vi "GUMSSequenceGenerator.vi"() -> ()   [LabVIEW 2011]
uses:
  gumLV8p2/D/Labviewsoft/transport/GUMS/Kelvinox drivers/ITCAPPS - Copie.LLB/ITCSignal.ctl
  gumLV8p2/D/Labviewsoft/transport/GUMS/Kelvinox drivers/ITCAPPS - Copie.LLB/ITCSignals.ctl
  DAC/Visa name1.vi
  GlobalVar.vi
  stopButton.vi
  monochromatorcontrol/perHandlemonochromator.vi
  users/nicolas/PHySpec-SDK-1.0.0/Labview-example/libPhyspec/libPhyspec.lvlib
panel:
  out "counter 2":i32
  out "DMMX":string[][](array[string])
  out "Bloop gen":u32
  out "WVlenloop gen":u32
  out "Tloop gen":u32
  out "loopchange":u32
  out "DACindic":bool
  in  "Gain Cluster 2":T1={"Vsd"="DAC 1", "I 2probe 2"="DMM1", "Vxy"="Lockin2 X", "Vxx"="DMM2", "I leak BG"="I K2400_01", "I leak TG"="I K2400_02", "I Gain 1"=1000000.0, "V Gain 1"=1.0, "conversion factor BG"=1.0, "Vin / Vout 1"=1.0, "V Gain 2"=1.0, "Vin / Vout 2"=1.0, "V Gain 3"=1.0, "Vin / Vout 3"=1.0, "I Gain 2"=1.0, "I Gain 3"=1.0, "V BG"="V K2400_01", "V TG"="V K2400_02", "conversion factor TG"=1.0, "Vin / Vout 4"=1.0, "Vin / Vout 5"=1.0, "Manual Gain 1"=1.0, "Manual Gain 2"=1.0, "Manual Gain 3"=1.0} {"conversion factor TG" items=["1 V/V"=1.0, "4 V/V"=4.0, "15 V/V"=15.0, "30 V/V"=30.0, "45 V/V"=45.0]; "I Gain 3" items=["1"=1.0, "10"=10.0, "100"=100.0, "1K"=1000.0, "10K"=10000.0, "100K"=100000.0, "1M"=1000000.0, "10M"=10000000.0, "100M"=100000000.0, "1G"=1000000000.0]; "I Gain 2" items=["1"=1.0, "10"=10.0, "100"=100.0, "1K"=1000.0, "10K"=10000.0, "100K"=100000.0, "1M"=1000000.0, "10M"=10000000.0, "100M"=100000000.0, "1G"=1000000000.0]; "V Gain 3" items=["1"=1.0, "10"=10.0, "100"=100.0, "1K"=1000.0, "10K"=10000.0]; "V Gain 2" items=["1"=1.0, "10"=10.0, "100"=100.0, "1K"=1000.0, "10K"=10000.0]; "conversion factor BG" items=["1 V/V"=1.0, "4 V/V"=4.0, "15 V/V"=15.0, "30 V/V"=30.0, "45 V/V"=45.0]; "V Gain 1" items=["1"=1.0, "10"=10.0, "100"=100.0, "1K"=1000.0, "10K"=10000.0]; "I Gain 1" items=["1"=1.0, "10"=10.0, "100"=100.0, "1K"=1000.0, "10K"=10000.0, "100K"=100000.0, "1M"=1000000.0, "10M"=10000000.0, "100M"=100000000.0, "1G"=1000000000.0]}
  in  "EmptyAllArrays":bool
  in  "Sweep back to zero":bool
  out "counter":i32
  out "Num elements in col":i32[](array[numeric])
  out "Current col":i32
  in  "Refresh Rate [ms]":i32=1000 min=0
  out "Current sweep":dbl
  out "ITC ref":T2={"ITC"=0, "Signal"=enum."Sensor 3"}
  in  "Cancel run":bool
  out "DAC":refnum<visa-resource-name>
  out "K2400 2":refnum<visa-resource-name>
  out "Lockin1":refnum<visa-resource-name>
  out "K2400 1":refnum<visa-resource-name>
  out "Total sweep sequence":dbl[][](array[numeric])
  in  "Device Cluster":T4={"K2400 1"="", "K2400_1"=FALSE, "K2400 2"="", "K2400_2"=FALSE, "Lockin1"="", "Lockin1 present"=FALSE, "Lockin2"="", "Lockin2 present"=FALSE, "TIC"="", "Tcontrol"="OFF", "DAC"="", "DAC present"=FALSE, "Bfield query"=FALSE, "Wvlen query"=FALSE, "ITC signal"={"ITC"=0, "Signal"=enum."Sensor 1"}, "DMMX"=[["DMM1", ""]]}
  in  "Tab Control":T5(tab)
  in  "Sweep Toothsaw":bool
  in  "Loop Cluster":T6
  in  "START":bool
  in  "genTotalSequence":bool
  out "row state":i32[](array[numeric])
  out "Priority type array":string[](array[string])
  out "TotalPnts":dbl
  in  "Sweep back\nto zero?":bool
  in  "Conversion Factor Fix\n1 V = ??":dbl=1.0
  in  "Fix type":string(combo)
  in  "Sweep Bias":dbl[](array[numeric])
  in  "Fix Bias":dbl[](array[numeric])
  in  "Priority sweep":i32=2
  in  "Priority fix":i32=2
  in  "sweep start [V]":dbl=-1.0 min=-200.0 max=200.0
  in  "sweep stop [V]":dbl=-5.0 min=-250.0 max=250.0
  in  "Nb steps":i32=800
  in  "sweep stop 2 [V]":dbl min=-250.0 max=250.0
  in  "Nb steps 2":i32
  in  "Nb Sweep":i32=1
  in  "Nb steps fix2":i32
  in  "Fix stop 2":dbl min=-250.0 max=250.0
  in  "Nb steps fix":i32=800
  in  "Fix stop":dbl=-5.0 min=-250.0 max=250.0
  in  "Fix start":dbl=-1.0 min=-200.0 max=200.0
  in  "genSweepArray":bool
  in  "genFixArray":bool
  in  "Sweep Instrument":string(combo)
  in  "Conversion Factor Sweep\n1 V = ??":dbl=1.0
  in  "Fix Instrument":string(combo)
  in  "Sweep type":string(combo)
  in  "V step K2400 [V]":dbl=0.001
  in  "genSweepArray sweeploop":bool
  in  "genfixArray fixlooop simple":bool
  in  "T [K]":dbl[](array[numeric])
  in  "Priority T":i32=2
  in  "Nb T steps":i32=800
  in  "T stop [K]":dbl=-1.0 min=-200.0 max=200.0
  in  "T start [K]":dbl=-1.0 min=-200.0 max=200.0
  in  "genTarray":bool
  in  "Add T points":bool
  in  "Zero ramp Rate [T/min] 2":dbl=0.2 min=-200.0 max=200.0
  in  "Sweep Field back to zero":bool
  in  "B [T]":dbl[](array[numeric])
  in  "Priority B":i32=2
  in  "B start [T]":dbl=-1.0 min=-200.0 max=200.0
  in  "B stop [T]":dbl=-1.0 min=-200.0 max=200.0
  in  "Sweep Rate [T/min]":dbl=0.1 min=-200.0 max=200.0
  in  "Nb B steps":i32=800
  in  "GenBarray":bool
  in  "Add B points":bool
  in  "Set Persistent":bool=TRUE
  in  "Power stabilization":bool=TRUE
  in  "Wvlen Start [nm]":dbl=400.0
  in  "Wavelength [nm]":dbl[](array[numeric])
  in  "genWVLEN array":bool
  in  "Add wvlen points":bool
  in  "Nb Wvlen steps":i32=350
  in  "Wvlen stop [nm]":dbl=1100.0
  out "Laser Power [W]":dbl format="%#.2g"
  in  "START FC":bool
  out "Field ok !":bool
  in  "Bipolar":bool
  in  "High T (K)":dbl
  in  "Temperature Up rate (K/min)":dbl
  in  "Waiting time (min)":dbl
  in  "Base T (K)":dbl
  in  "sweep rate B (T/min)":dbl
  in  "Cooling field (T)":dbl
  out "I am":string
  in  "File Basename":string
  out "Bias factor":dbl
  in  "SD bias [V]":dbl=-1.0 min=-200.0 max=200.0
  in  "Nb steps Increase 2":dbl=10.0
  in  "Gate Increase 2 (V)":dbl=0.1
  in  "Nb steps Increase":dbl=10.0
  in  "Gate Increase (V)":dbl=-0.1
  out "x .or. y?":bool
  in  "Step Delay (ms)":dbl=1000.0
  out "Total Progress":dbl(slide) scale=0.0..1.0
  in  "Nb Loop":i32
  out "Nb Loop Indicator":i32=2
  out "Nb Sweep Indicator":i32=3
  out "conversion factor sweep":dbl(ring)=1.0 items=["1 V/V"=1.0, "4 V/V"=4.0, "15 V/V"=15.0, "30 V/V"=30.0, "45 V/V"=45.0]
  in  "stop":bool
  in  "V step [V]":dbl=0.001
  in  "Folder Name":path=path "D:/users/marc/20180122_LiIon_EL/Freezing02/OutputHighT002p2.dat"
  # "Magnetic Field"
  # "Wavelength"
  # "IV Sweep Setting"
  # "IV Fix Setting"
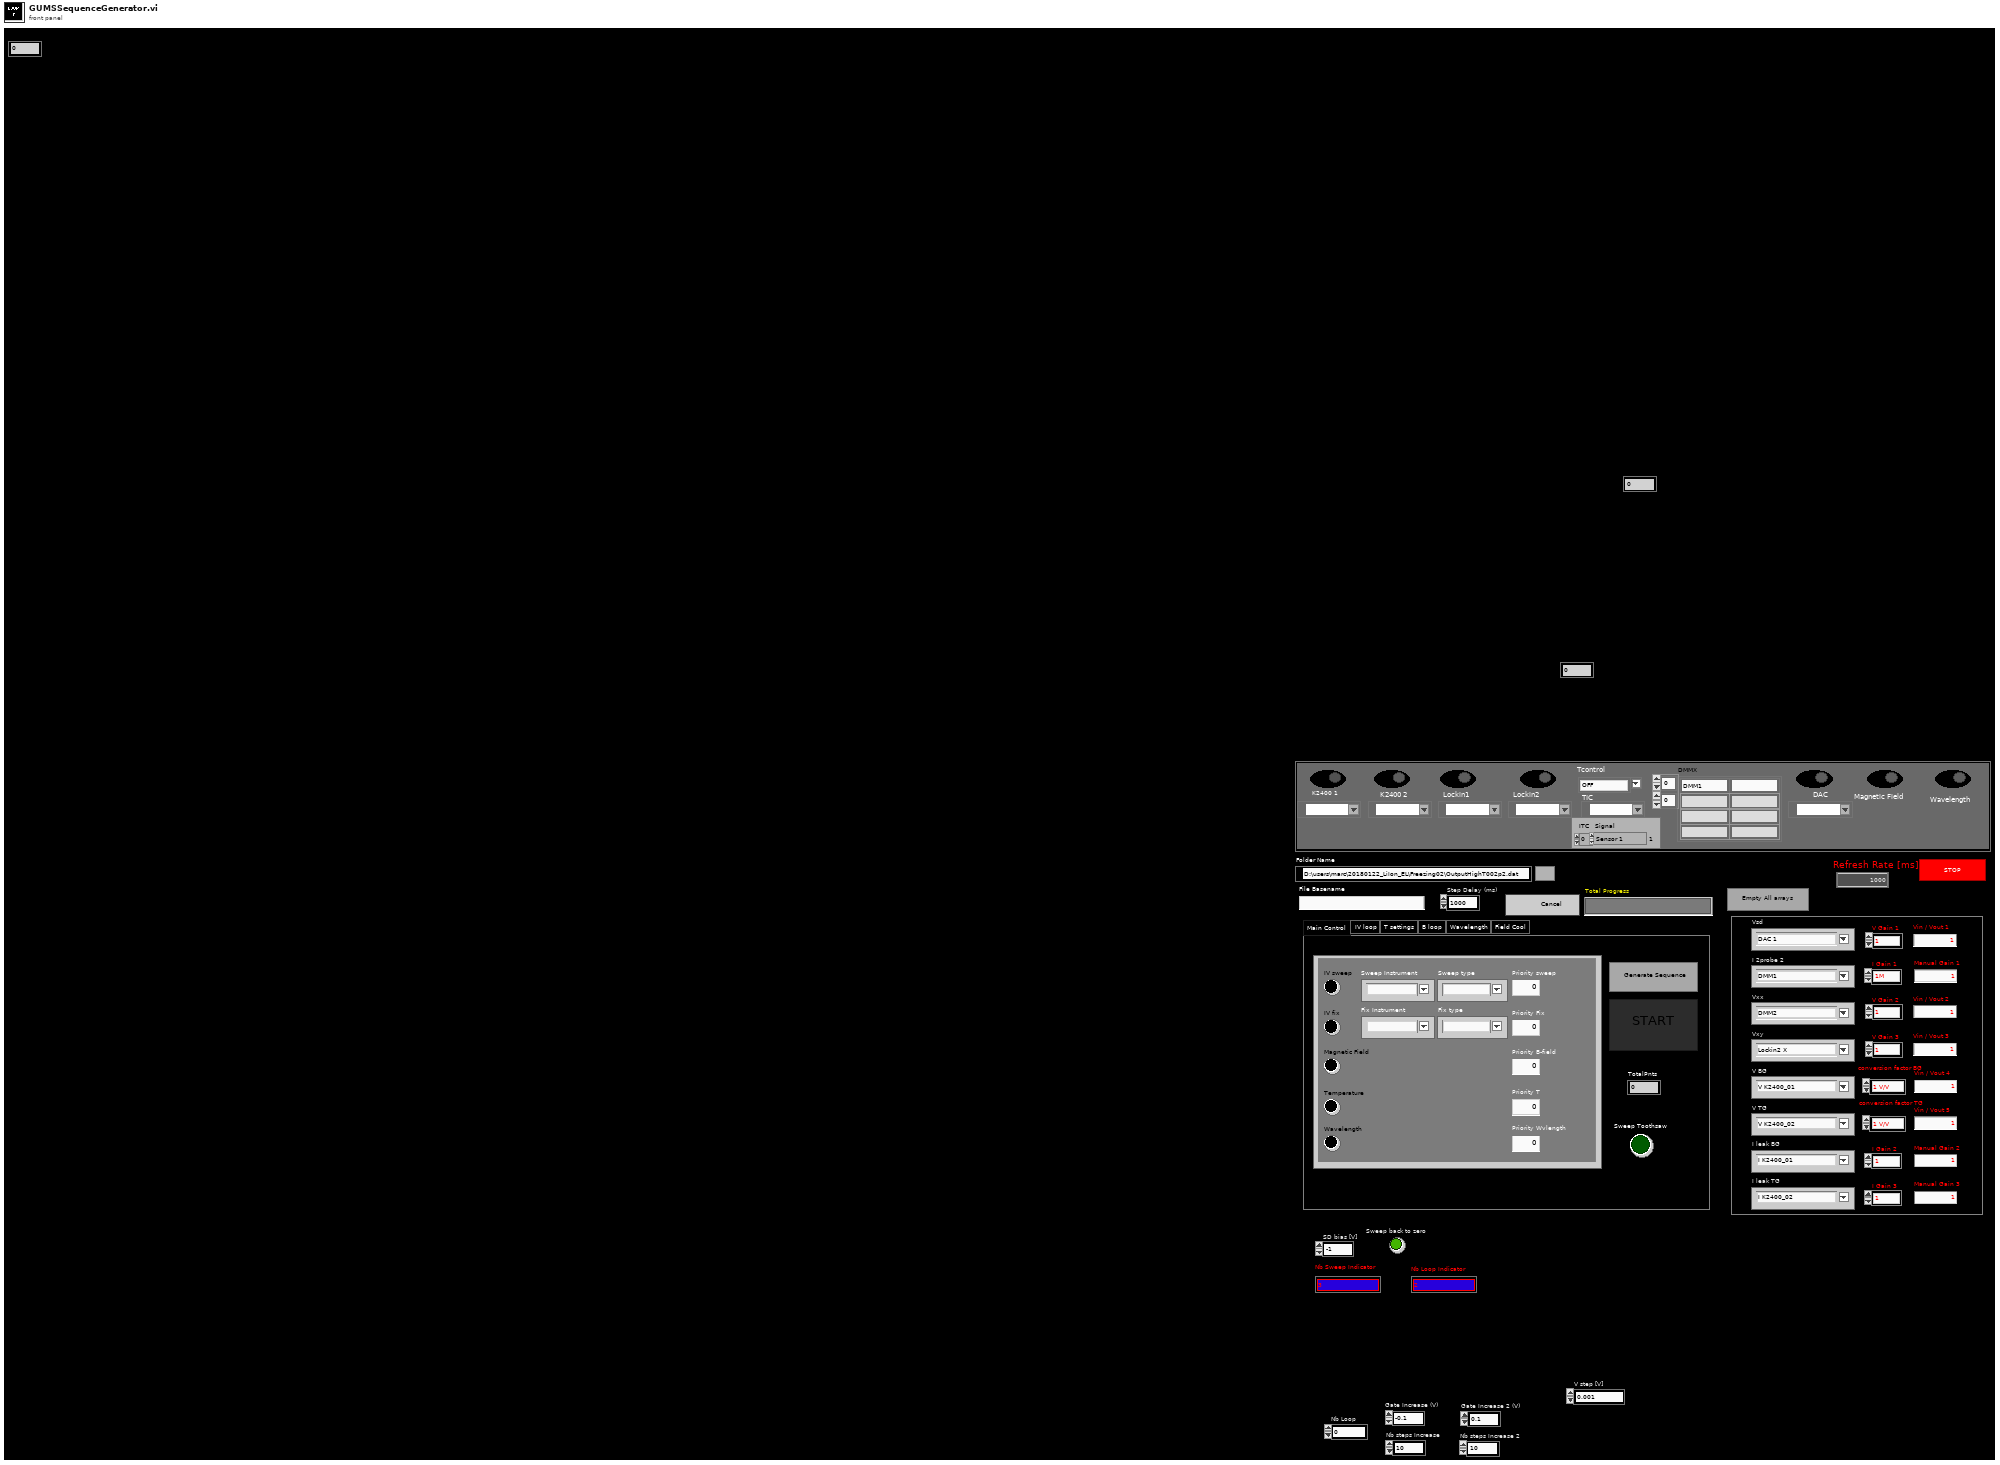
[diagram p1: front panel]
types:
  T1 = cluster{"Vsd":string, "I 2probe 2":string, "Vxy":string, "Vxx":string, "I leak BG":string, "I leak TG":string, "I Gain 1":dbl, "V Gain 1":dbl, "conversion factor BG":dbl, "Vin / Vout 1":dbl, "V Gain 2":dbl, "Vin / Vout 2":dbl, "V Gain 3":dbl, "Vin / Vout 3":dbl, "I Gain 2":dbl, "I Gain 3":dbl, "V BG":string, "V TG":string, "conversion factor TG":dbl, "Vin / Vout 4":dbl, "Vin / Vout 5":dbl, "Manual Gain 1":dbl, "Manual Gain 2":dbl, "Manual Gain 3":dbl}
  T2 = typedef "ITCSignal.ctl" = cluster{"ITC":u16, "Signal":T3}
  T3 = typedef "ITCSignals.ctl" = enum16{"Setpoint", "Sensor 1", "Sensor 2", "Sensor 3", "Needle Valve %", "Heater %"}
  T4 = cluster{"K2400 1":refnum<visa-resource-name>, "K2400_1":bool, "K2400 2":refnum<visa-resource-name>, "K2400_2":bool, "Lockin1":refnum<visa-resource-name>, "Lockin1 present":bool, "Lockin2":refnum<visa-resource-name>, "Lockin2 present":bool, "TIC":refnum<visa-resource-name>, "Tcontrol":string, "DAC":refnum<visa-resource-name>, "DAC present":bool, "Bfield query":bool, "Wvlen query":bool, "ITC signal":T2, "DMMX":string[][]}
  T5 = enum32{"Main Control", "IV loop", "T settings", "B loop", "Wavelength", "Field Cool"}
  T6 = cluster{"Sweep Instrument":string, "Sweep type":string, "Fix Instrument":string, "Fix type":string, "IV sweep":bool, "IV fix":bool, "Magnetic Field":bool, "Temperature":bool, "Wavelength":bool, "Priority sweep":dbl, "Priority Fix":dbl, "Priority B-field":dbl, "Priority T":dbl, "Priority Wvlength":dbl}
  T7 = cluster{"Power Stabilization":bool, "Laser Power [W]":dbl, "Power precision":dbl}
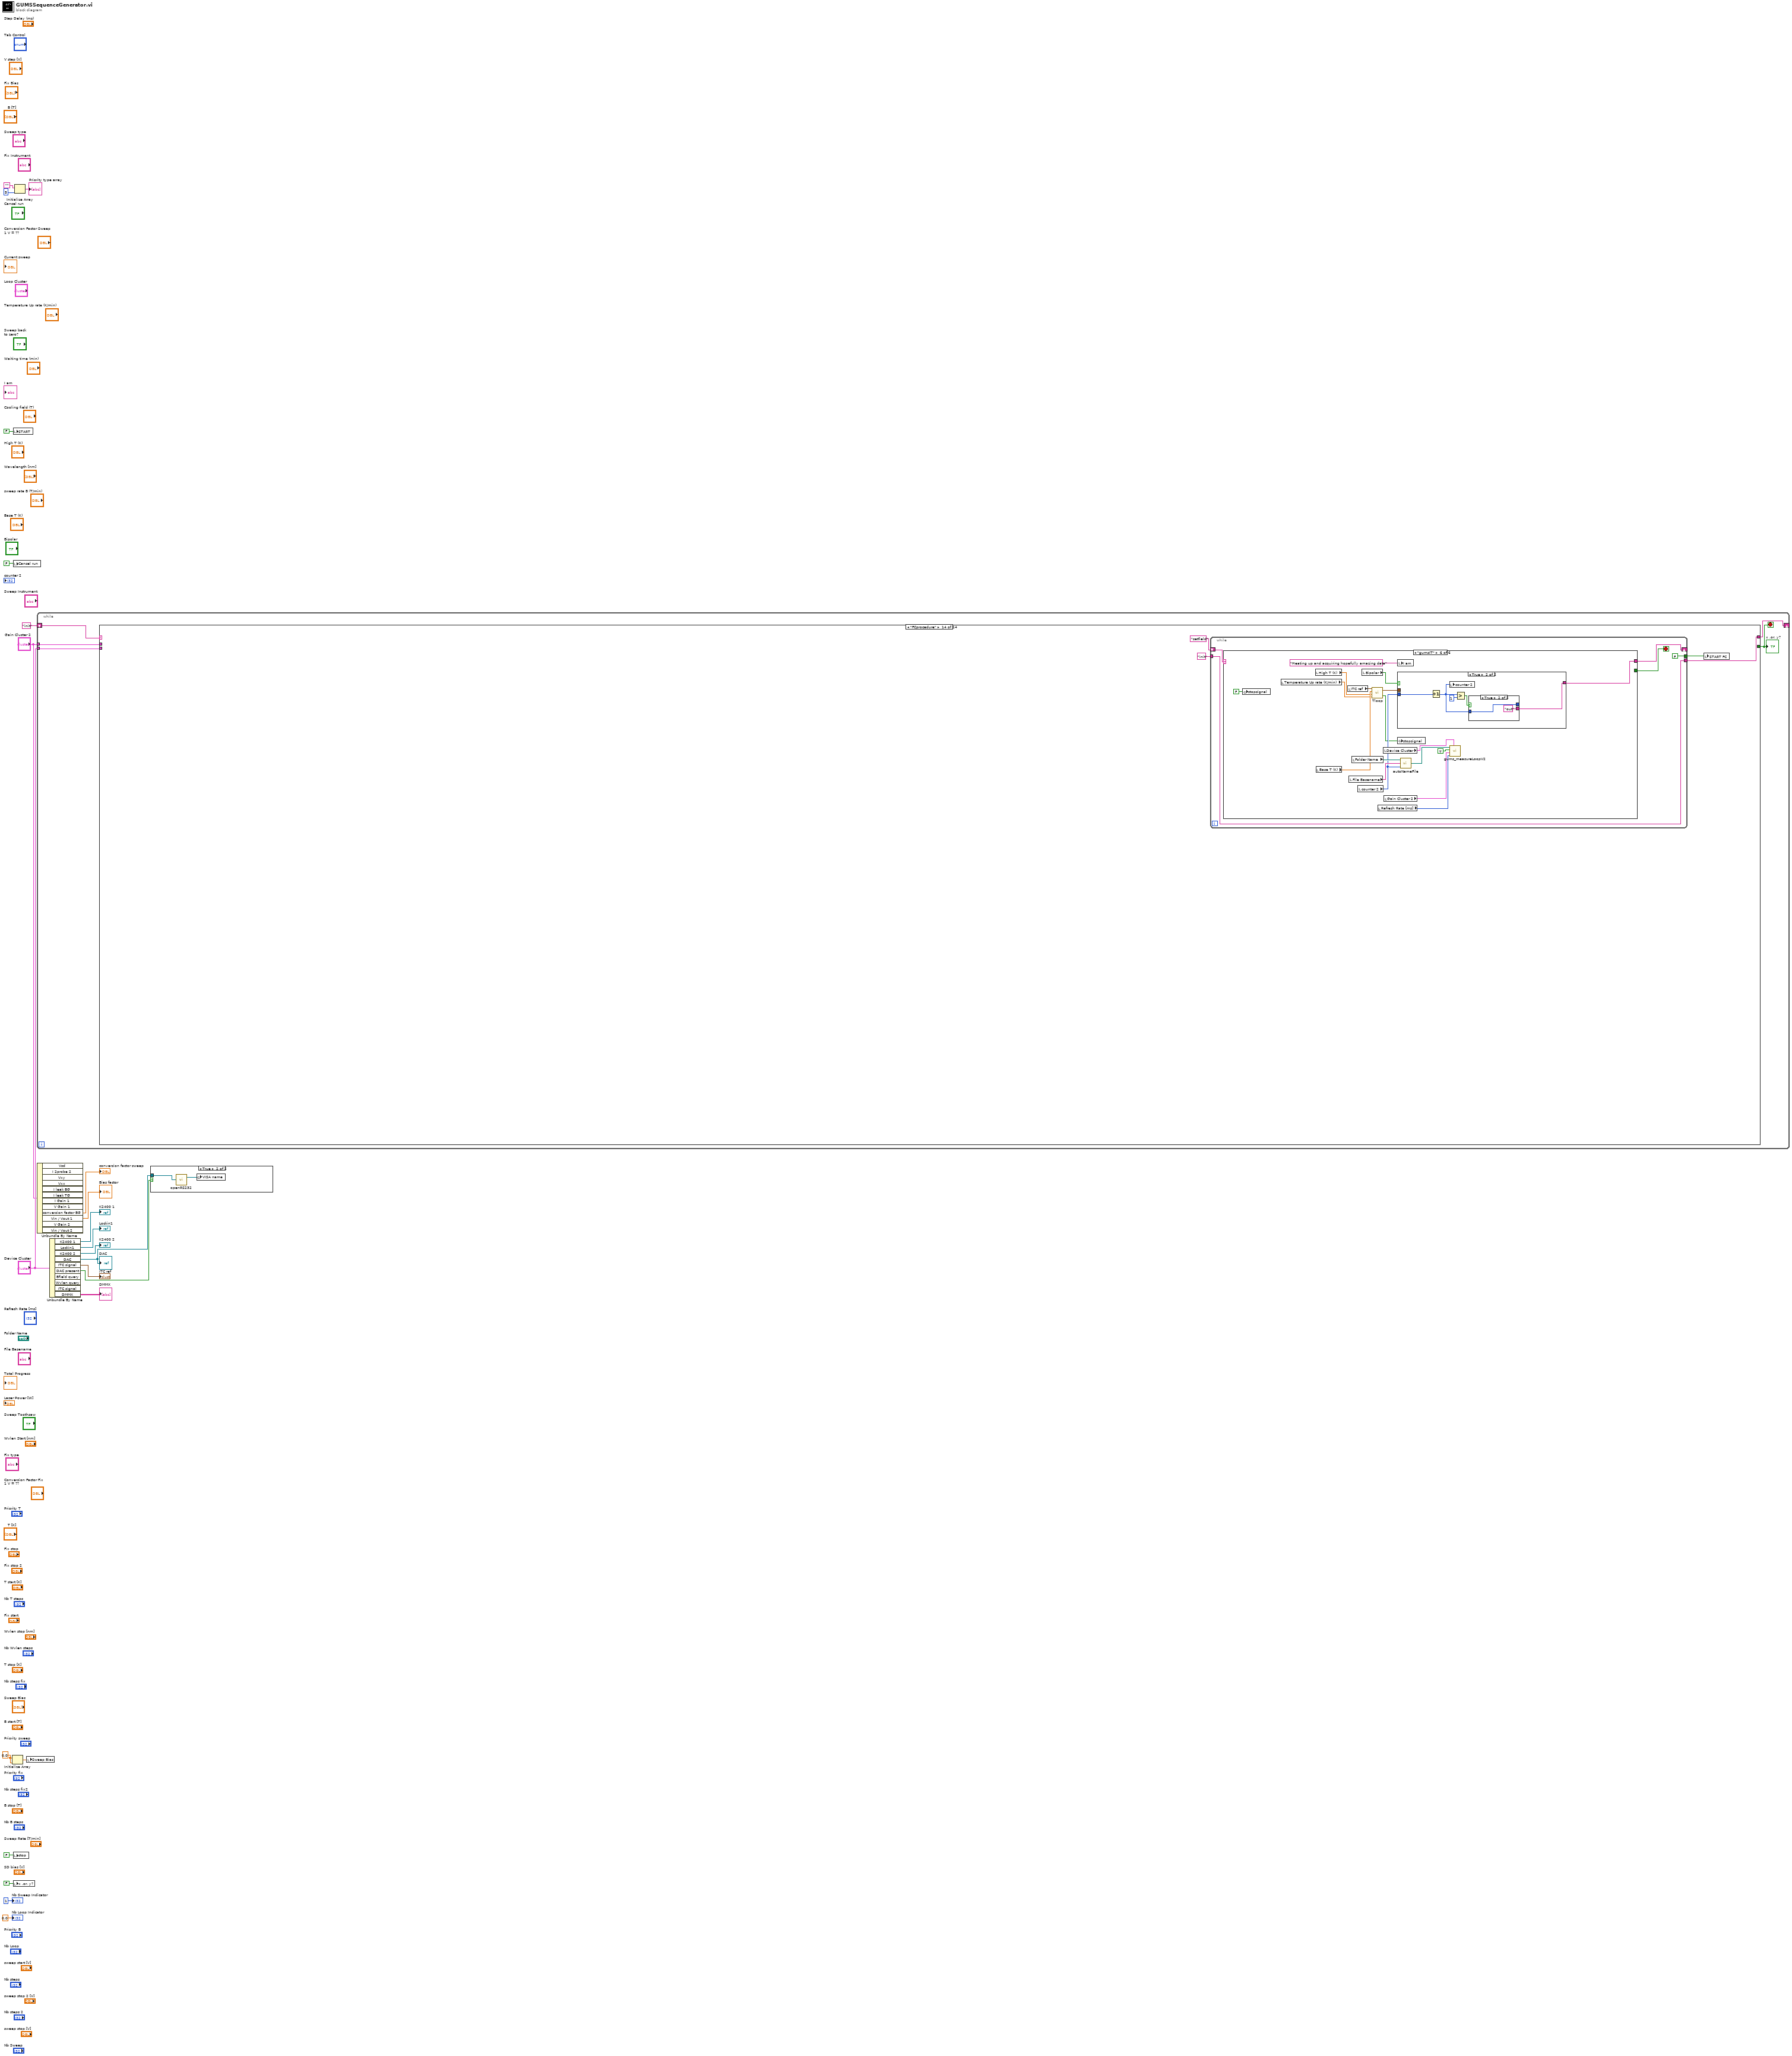
[diagram p0: block diagram]
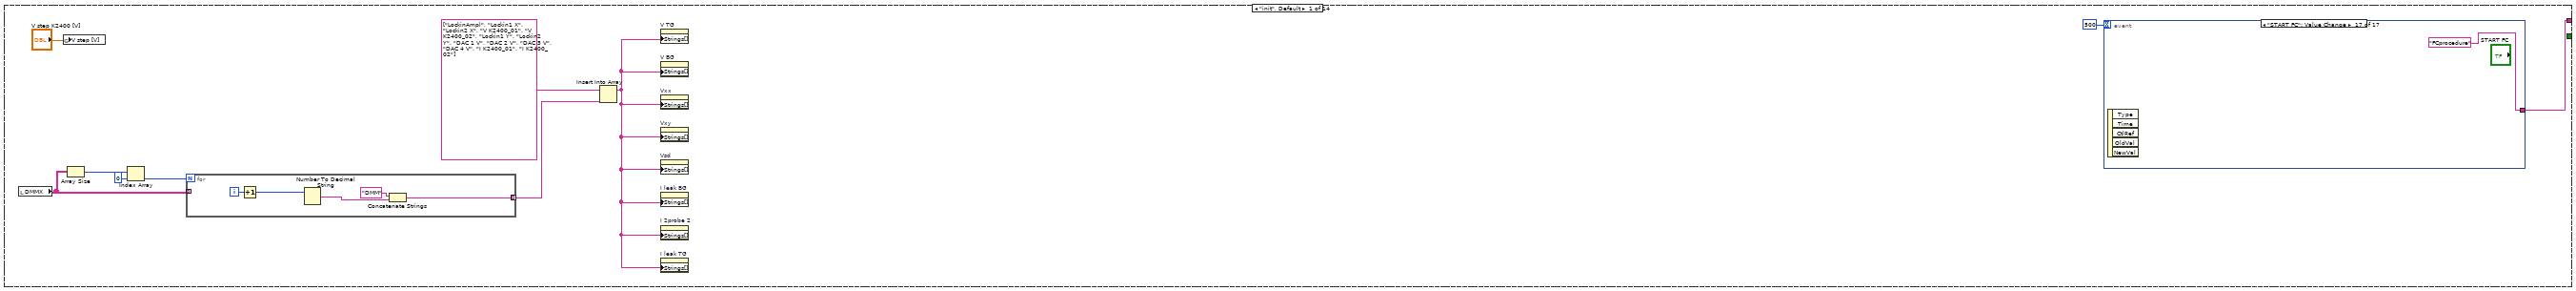
[diagram p3: hidden frame]
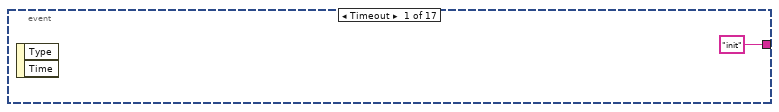
[diagram p4: hidden frame]
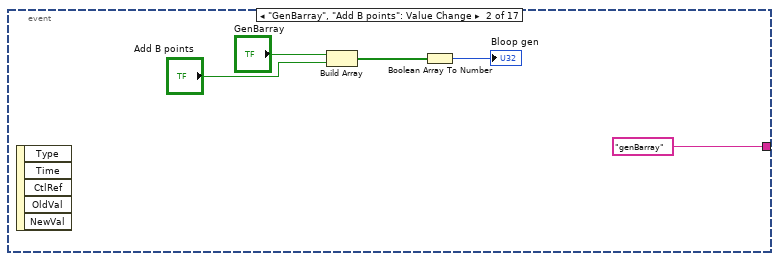
[diagram p5: hidden frame]
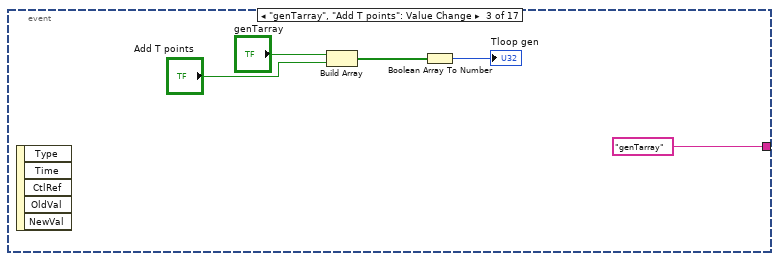
[diagram p6: hidden frame]
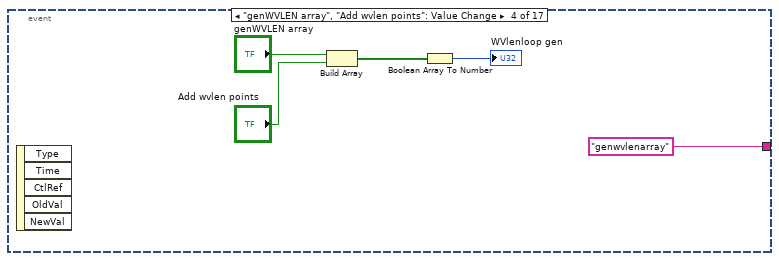
[diagram p7: hidden frame]
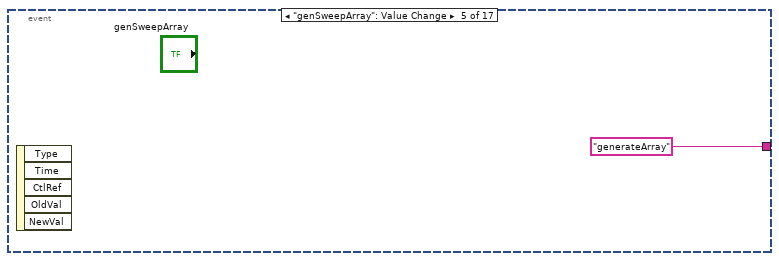
[diagram p8: hidden frame]
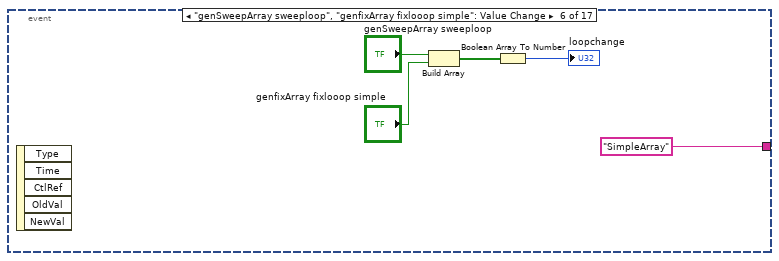
[diagram p9: hidden frame]
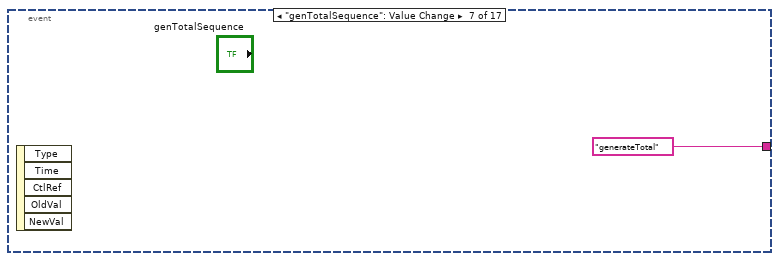
[diagram p10: hidden frame]
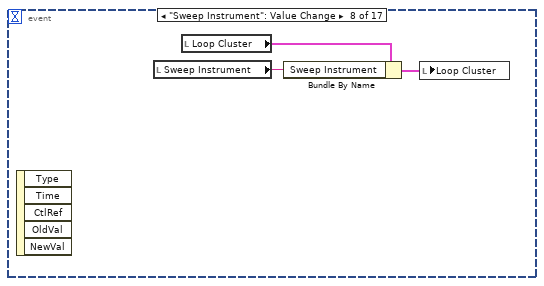
[diagram p11: hidden frame]
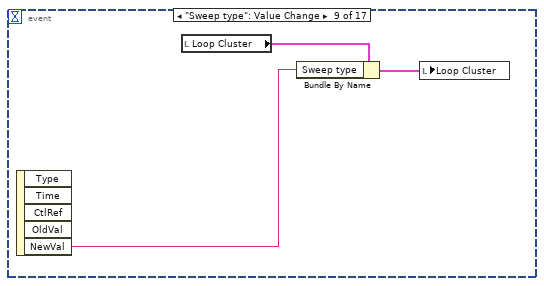
[diagram p12: hidden frame]
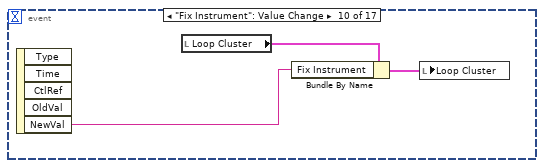
[diagram p13: hidden frame]
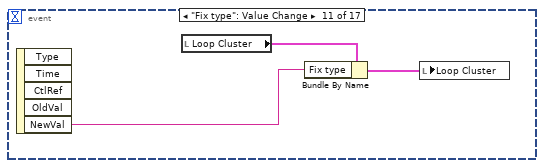
[diagram p14: hidden frame]
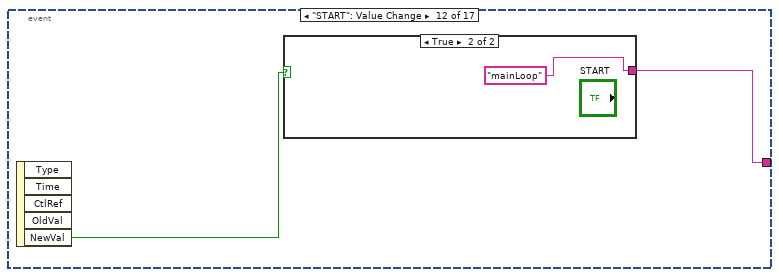
[diagram p15: hidden frame]
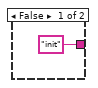
[diagram p16: hidden frame]
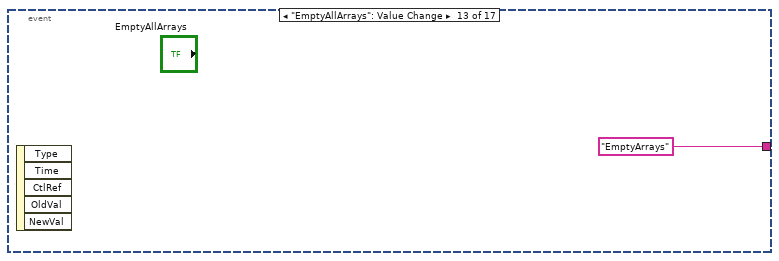
[diagram p17: hidden frame]
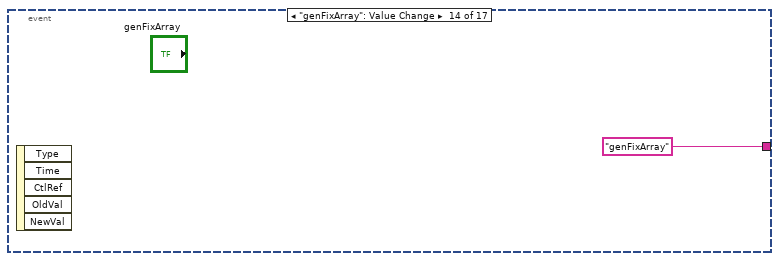
[diagram p18: hidden frame]
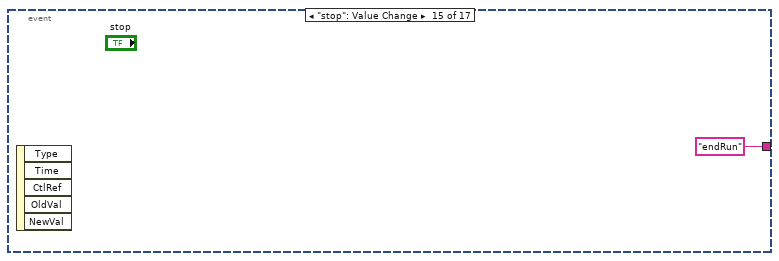
[diagram p19: hidden frame]
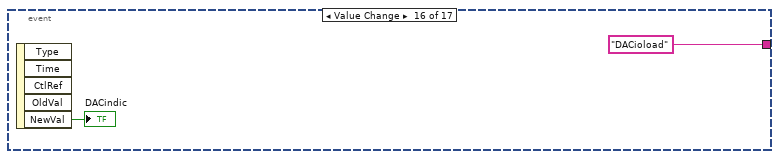
[diagram p20: hidden frame]
diagram:
  w6 = 0.0
  n1 = Initialize Array(w6, w6) -> (w7:dbl[])
  n2 = local write "START"(FALSE ("START")) -> ()
  n3 = local write "Cancel run"(FALSE ("Cancel run")) -> ()
  n4 = local write "stop"(FALSE ("stop")) -> ()
  n5 = local write "x .or. y?"(FALSE ("x .or. y?")) -> ()
  n6 = Initialize Array("", 5 ("dimension size")) -> (→"Priority type array":string[])
  n7 = local write "Sweep Bias"(w7) -> ()
  n8 = while {
    shift-right: [w24] -> _
    shift-left: "init" -> [w28]
    tunnel: "Gain Cluster 2" -> [w26]
    tunnel: "Device Cluster" -> [w25]
    stop <- w27 stop-if-true
    n9 = case shown="\"FCprocedure\"" w28 {
      tunnel: [_ _ _ _ _ _ _ _ _ _ TRUE _ _ _] -> w27
      tunnel: [w37 "init" "init" "init" "init" "init" "init" "init" w264 "generateArray" "" "init" w558 w567] -> w24
      tunnel: w26 -> [_ _ _ _ _ _ _ _ _ _ _ _ _ _]
      tunnel: w25 -> [_ _ _ _ _ _ _ _ _ _ _ _ _ _]
      frame "init", Default {
        n10 = local read "DMMX"() -> (w31:string[][])
        n11 = global write "GlobalVar.vi" "V step [V]"("V step K2400 [V]") -> ()
        n12 = Array Size(array=w31) -> (size(s)=w34:i32[])
        n13 = Index Array(array=w34, index=0) -> (element=w33:i32)
        n14 = for {
          N: w33 -> [_]
          tunnel: w31 -> [_] mode=indexing
          tunnel: [w39] -> w30 mode=indexing
          i -> [w42]
          n15 = Increment(x=w42) -> (x+1=w40:i32)
          n16 = Number To Decimal String(number=w40) -> (decimal integer string=w41:string)  [unwired: 1 in]
          n17 = Concatenate Strings("DMM", w41) -> (w39:string)
        }
        n18 = Insert Into Array(array=string[] ["LockinAmpl", "Lockin1 X", "Lockin2 X", "V K2400_01", "V K2400_02", "Lockin1 Y", "Lockin2 Y", "DAC 1 V", "DAC 2 V", "DAC 3 V", "DAC 4 V", "I K2400_01", "I K2400_02"] ("Strings []"), new element=w30) -> (w29:string[])  [unwired: 1 in]
        n19 = property on="V TG" class="CmbBox"("Strings[]"=w29) -> ()  [unwired: 2 in, 2 out]
        n20 = property on="V BG" class="CmbBox"("Strings[]"=w29) -> ()  [unwired: 2 in, 2 out]
        n21 = property on="Vxx" class="CmbBox"("Strings[]"=w29) -> ()  [unwired: 2 in, 2 out]
        n22 = property on="Vxy" class="CmbBox"("Strings[]"=w29) -> ()  [unwired: 2 in, 2 out]
        n23 = property on="Vsd" class="CmbBox"("Strings[]"=w29) -> ()  [unwired: 2 in, 2 out]
        n24 = property on="I leak BG" class="CmbBox"("Strings[]"=w29) -> ()  [unwired: 2 in, 2 out]
        n25 = property on="I 2probe 2" class="CmbBox"("Strings[]"=w29) -> ()  [unwired: 2 in, 2 out]
        n26 = property on="I leak TG" class="CmbBox"("Strings[]"=w29) -> ()  [unwired: 2 in, 2 out]
        n27 = event shown="[16] \"START FC\": Value Change" {
          selector: _ -> [_ _ _ _ _ _ _ _ _ _ _ _ _ _ _ _ _]
          dyn-events: _ -> [_ _ _ _ _ _ _ _ _ _ _ _ _ _ _ _ _]
          timeout: 500 -> [_ _ _ _ _ _ _ _ _ _ _ _ _ _ _ _ _]
          tunnel: ["init" "genBarray" "genTarray" "genwvlenarray" "generateArray" "SimpleArray" "generateTotal" _ _ _ _ w79 "EmptyArrays" "genFixArray" "endRun" "DACioload" "FCprocedure"] -> w37
          event Timeout {
            n28 = event-data() -> ()  [unwired: 1 in, 2 out]
          }
          event "GenBarray", "Add B points": Value Change {
            n29 = event-data() -> ()  [unwired: 1 in, 5 out]
            n30 = Build Array("GenBarray", "Add B points") -> (w48:bool[])
            n31 = Boolean Array To Number(Boolean array=w48) -> (number=→"Bloop gen":u32)
          }
          event "genTarray", "Add T points": Value Change {
            n32 = event-data() -> ()  [unwired: 1 in, 5 out]
            n33 = Build Array("genTarray", "Add T points") -> (w53:bool[])
            n34 = Boolean Array To Number(Boolean array=w53) -> (number=→"Tloop gen":u32)
          }
          event "genWVLEN array", "Add wvlen points": Value Change {
            n35 = event-data() -> ()  [unwired: 1 in, 5 out]
            n36 = Build Array("genWVLEN array", "Add wvlen points") -> (w58:bool[])
            n37 = Boolean Array To Number(Boolean array=w58) -> (number=→"WVlenloop gen":u32)
          }
          event "genSweepArray": Value Change {
            n38 = event-data() -> ()  [unwired: 1 in, 5 out]
          }
          event "genSweepArray sweeploop", "genfixArray fixlooop simple": Value Change {
            n39 = event-data() -> ()  [unwired: 1 in, 5 out]
            n40 = Build Array("genSweepArray sweeploop", "genfixArray fixlooop simple") -> (w62:bool[])
            n41 = Boolean Array To Number(Boolean array=w62) -> (number=→"loopchange":u32)
          }
          event "genTotalSequence": Value Change {
            n42 = event-data() -> ()  [unwired: 1 in, 5 out]
          }
          event "Sweep Instrument": Value Change {
            n43 = event-data() -> ()  [unwired: 1 in, 5 out]
            n44 = local read "Sweep Instrument"() -> (w68:string)
            n45 = local read "Loop Cluster"() -> (w69:T6)
            n46 = Bundle By Name(cluster=w69, "Sweep Instrument"=w68) -> (w67:T6)
            n47 = local write "Loop Cluster"(w67) -> ()
          }
          event "Sweep type": Value Change {
            n48 = event-data() -> ("NewVal"=w70:string)  [unwired: 1 in, 4 out]
            n49 = local read "Loop Cluster"() -> (w72:T6)
            n50 = Bundle By Name(cluster=w72, "Sweep type"=w70) -> (w71:T6)
            n51 = local write "Loop Cluster"(w71) -> ()
          }
          event "Fix Instrument": Value Change {
            n52 = event-data() -> ("NewVal"=w73:string)  [unwired: 1 in, 4 out]
            n53 = local read "Loop Cluster"() -> (w74:T6)
            n54 = Bundle By Name(cluster=w74, "Fix Instrument"=w73) -> (w75:T6)
            n55 = local write "Loop Cluster"(w75) -> ()
          }
          event "Fix type": Value Change {
            n56 = event-data() -> ("NewVal"=w78:string)  [unwired: 1 in, 4 out]
            n57 = local read "Loop Cluster"() -> (w77:T6)
            n58 = Bundle By Name(cluster=w77, "Fix type"=w78) -> (w76:T6)
            n59 = local write "Loop Cluster"(w76) -> ()
          }
          event "START": Value Change {
            n60 = event-data() -> ("NewVal"=w80:bool)  [unwired: 1 in, 4 out]
            n61 = case shown="True" w80 {
              tunnel: ["init" "mainLoop"] -> w79
              frame False {
              }
              frame True {
              }
            }
          }
          event "EmptyAllArrays": Value Change {
            n62 = event-data() -> ()  [unwired: 1 in, 5 out]
          }
          event "genFixArray": Value Change {
            n63 = event-data() -> ()  [unwired: 1 in, 5 out]
          }
          event "stop": Value Change {
            n64 = event-data() -> ()  [unwired: 1 in, 5 out]
          }
          event "Device Cluster.DAC present": Value Change {
            n65 = event-data() -> ("NewVal"=→"DACindic":bool)  [unwired: 1 in, 4 out]
          }
          event "START FC": Value Change {
            n66 = event-data() -> ()  [unwired: 1 in, 5 out]
          }
        }
      }
      frame "SimpleArray" {
        n67 = local read "loopchange"() -> (w89:u32)
        n68 = case shown="2" w89 {
          frame 0, Default {
          }
          frame 1 {
            n69 = local read "sweep start [V]"() -> (w91:dbl)
            n70 = local read "sweep stop [V]"() -> (w92:dbl)
            n71 = local read "Nb steps"() -> (w93:i32)
            n72 = call "createSimpleArray.vi"("nbpoint1"=w93, "Bgstop"=w92, "Bgstart"=w91) -> ("Outarray"=w94:dbl[])
            n73 = local write "Sweep Bias"(w94) -> ()
          }
          frame 2 {
            n74 = local read "Nb steps fix"() -> (w95:i32)
            n75 = local read "Fix start"() -> (w97:dbl)
            n76 = local read "Fix stop"() -> (w96:dbl)
            n77 = call "createSimpleArray.vi"("nbpoint1"=w95, "Bgstop"=w96, "Bgstart"=w97) -> ("Outarray"=w98:dbl[])
            n78 = local write "Fix Bias"(w98) -> ()
          }
        }
      }
      frame "generateTotal" {
        n79 = local read "Loop Cluster"() -> (w107:T6)
        n80 = Unbundle By Name(w107) -> ("IV sweep"=w127:bool, "IV fix"=w126:bool, "Magnetic Field"=w125:bool, "Temperature"=w124:bool, "Wavelength"=w123:bool, "Priority sweep"=w118:dbl, "Priority Fix"=w117:dbl, "Priority B-field"=w116:dbl, "Priority T"=w115:dbl, "Priority Wvlength"=w110:dbl)
        n81 = Build Array(w127, w126, w125, w124, w123) -> (w121:bool[])
        n82 = Decrement(x=w118) -> (x-1=w111:dbl)
        n83 = Decrement(x=w117) -> (x-1=w112:dbl)
        n84 = Decrement(x=w116) -> (x-1=w113:dbl)
        n85 = Decrement(x=w115) -> (x-1=w114:dbl)
        n86 = Decrement(x=w110) -> (x-1=w109:dbl)
        n87 = Boolean To (0,1)(Boolean=w121) -> (0, 1=w122:i16[])
        n88 = Add Array Elements(numeric array=w122) -> (sum=w120:i16)
        n89 = for {
          N: w120 -> [_]
          shift-right: [w152] -> w102
          shift-left: dbl[][] [] ("Array In") -> [w153]
          tunnel: w114 -> [w149]
          tunnel: w113 -> [w150]
          tunnel: w112 -> [w151]
          tunnel: w111 -> [w143]
          tunnel: w109 -> [w145]
          shift-right: [w138] -> w106
          shift-left: string[] [] -> [w136]
          i -> [w146]
          n90 = Equal?(x=w143, y=w146) -> (x = y?=w142:bool)
          n91 = Equal?(x=w151, y=w146) -> (x = y?=w141:bool)
          n92 = Equal?(x=w150, y=w146) -> (x = y?=w140:bool)
          n93 = Equal?(x=w149, y=w146) -> (x = y?=w139:bool)
          n94 = Equal?(x=w145, y=w146) -> (x = y?=w144:bool)
          n95 = Build Array(w142, w141, w140, w139, w144) -> (w148:bool[])
          n96 = Boolean Array To Number(Boolean array=w148) -> (number=w147:u32)
          n97 = case shown="16" w147 {
            tunnel: [_ "sweeparray" "Fixarray" "Bfield" ("Fix Instrument") "Temperature" "wavelength"] -> w137
            tunnel: [_ w155 w157 w158 w160 w162] -> w135
            frame 0, Default {
            }
            frame 1 {
              n98 = local read "Sweep Bias"() -> (w155:dbl[])
            }
            frame 2 {
              n99 = local read "Fix Bias"() -> (w157:dbl[])
            }
            frame 4 {
              n100 = local read "B [T]"() -> (w158:dbl[])
            }
            frame 8 {
              n101 = local read "T [K]"() -> (w160:dbl[])
            }
            frame 16 {
              n102 = local read "Wavelength [nm]"() -> (w162:dbl[])
            }
          }
          n103 = call "generateFinalArray.vi"("new array"=w135, "Array In"=w153) -> ("Array out"=w152:dbl[][])
          n104 = Build Array (concatenate)(w136, w137) -> (w138:string[])
        }
        "Total sweep sequence" <- w102
        n105 = local write "Priority type array"(w106) -> ()
        n106 = Index Array(array=w102, index (row)=0) -> (element=w99:dbl[])  [unwired: 1 in]
        n107 = Array Size(array=w99) -> (size(s)=w101:i32)
        n108 = Decrement(x=w101) -> (x-1=w100:i32)
        n109 = for {
          N: w100 -> [_]
          tunnel: w99 -> [w132]
          shift-right: [w129] -> w105
          shift-left: 1 ("index") -> [w130]
          i -> [w134]
          n110 = Increment(x=w134) -> (x+1=w133:i32)
          n111 = Index Array(array=w132, index=w133) -> (element=w131:dbl)
          n112 = Multiply(x=w130, y=w131) -> (x*y=w129:dbl)
        }
        n113 = local write "TotalPnts"(w105) -> ()
      }
      frame "generateArray" {
        w165 = 0.0 ("element")
        n114 = local read "Nb Sweep"() -> (w172:i32)
        n115 = local read "Priority sweep"() -> (w166:i32)
        n116 = Initialize Array(w165, w165) -> (w164:dbl[])
        n117 = local read "Priority type array"() -> (w170:string[])
        n118 = for {
          N: w172 -> [_]
          shift-right: [w176] -> w171
          shift-left: w164 -> [w175]
          n119 = local read "sweep stop 2 [V]"() -> (w178:dbl)
          n120 = local read "sweep stop [V]"() -> (w177:dbl)
          n121 = local read "sweep start [V]"() -> (w179:dbl)
          n122 = local read "Nb steps 2"() -> (w180:i32)
          n123 = local read "Nb steps"() -> (w181:i32)
          n124 = call "createLoopArray.vi"("Bgstop"=w177, "Bgstop2"=w178, "nbpoint1"=w181, "nbpoint2"=w180, "Bgstart"=w179) -> ("Outarray"=w174:dbl[])
          n125 = Build Array (concatenate)(w175, w174) -> (w176:dbl[])
        }
        n126 = Decrement(x=w166) -> (x-1=w167:i32)
        n127 = Replace Array Subset(array=w170, new element="sweeparray" ("new element/subarray"), index=w167) -> (w169:string[])
        n128 = local write "Priority type array"(w169) -> ()
        n129 = local write "Sweep Bias"(w171) -> ()
      }
      frame "genFixArray" {
        n130 = local read "Priority fix"() -> (w182:i32)
        n131 = local read "Nb Sweep"() -> (w189:i32)
        n132 = local read "Fix Bias"() -> (w188:dbl[])
        n133 = local read "Priority type array"() -> (w186:string[])
        n134 = for {
          N: w189 -> [_]
          shift-right: [w193] -> w187
          shift-left: w188 -> [w192]
          n135 = local read "Nb steps fix2"() -> (w197:i32)
          n136 = local read "Nb steps fix"() -> (w198:i32)
          n137 = local read "Fix stop 2"() -> (w195:dbl)
          n138 = local read "Fix start"() -> (w196:dbl)
          n139 = local read "Fix stop"() -> (w194:dbl)
          n140 = call "createLoopArray.vi"("Bgstop"=w194, "Bgstop2"=w195, "nbpoint1"=w198, "nbpoint2"=w197, "Bgstart"=w196) -> ("Outarray"=w191:dbl[])
          n141 = Build Array (concatenate)(w192, w191) -> (w193:dbl[])
        }
        n142 = Decrement(x=w182) -> (x-1=w183:i32)
        n143 = Replace Array Subset(array=w186, new element="Fixarray" ("new element/subarray"), index=w183) -> (w185:string[])
        n144 = local write "Priority type array"(w185) -> ()
        n145 = local write "Fix Bias"(w187) -> ()
      }
      frame "genTarray" {
        n146 = local read "Nb T steps"() -> (w201:i32)
        n147 = local read "Tloop gen"() -> (w204:u32)
        n148 = local read "T start [K]"() -> (w203:dbl)
        n149 = local read "T stop [K]"() -> (w202:dbl)
        n150 = local read "T [K]"() -> (w200:dbl[])
        n151 = case shown="2" w204 {
          tunnel: w203 -> [_ w210 w216]
          tunnel: w202 -> [_ w209 w215]
          tunnel: w201 -> [_ w208 w214]
          tunnel: [w206 w207 w211] -> w199
          tunnel: w200 -> [w206 _ w213]
          frame 0, Default {
          }
          frame 1 {
            n152 = call "createSimpleArray.vi"("nbpoint1"=w208, "Bgstop"=w209, "Bgstart"=w210) -> ("Outarray"=w207:dbl[])
          }
          frame 2 {
            n153 = call "createSimpleArray.vi"("nbpoint1"=w214, "Bgstop"=w215, "Bgstart"=w216) -> ("Outarray"=w212:dbl[])
            n154 = Insert Into Array(array=w213, new element=w212) -> (w211:dbl[])  [unwired: 1 in]
          }
        }
        n155 = local write "T [K]"(w199) -> ()
      }
      frame "genBarray" {
        n156 = local read "Nb B steps"() -> (w219:i32)
        n157 = local read "Bloop gen"() -> (w222:u32)
        n158 = local read "B start [T]"() -> (w221:dbl)
        n159 = local read "B stop [T]"() -> (w220:dbl)
        n160 = local read "B [T]"() -> (w218:dbl[])
        n161 = case shown="2" w222 {
          tunnel: w221 -> [_ w228 w234]
          tunnel: w220 -> [_ w227 w233]
          tunnel: w219 -> [_ w226 w232]
          tunnel: [w224 w225 w229] -> w217
          tunnel: w218 -> [w224 _ w231]
          frame 0, Default {
          }
          frame 1 {
            n162 = call "createSimpleArray.vi"("nbpoint1"=w226, "Bgstop"=w227, "Bgstart"=w228) -> ("Outarray"=w225:dbl[])
          }
          frame 2 {
            n163 = call "createSimpleArray.vi"("nbpoint1"=w232, "Bgstop"=w233, "Bgstart"=w234) -> ("Outarray"=w230:dbl[])
            n164 = Insert Into Array(array=w231, new element=w230) -> (w229:dbl[])  [unwired: 1 in]
          }
        }
        n165 = local write "B [T]"(w217) -> ()
      }
      frame "genwvlenarray" {
        n166 = local read "Wavelength [nm]"() -> (w236:dbl[])
        n167 = local read "Wvlen Start [nm]"() -> (w239:dbl)
        n168 = local read "Wvlen stop [nm]"() -> (w238:dbl)
        n169 = local read "Nb Wvlen steps"() -> (w237:i32)
        n170 = local read "WVlenloop gen"() -> (w240:u32)
        n171 = case shown="2" w240 {
          tunnel: w239 -> [_ w246 w252]
          tunnel: w238 -> [_ w245 w251]
          tunnel: w237 -> [_ w244 w250]
          tunnel: [w242 w243 w247] -> w235
          tunnel: w236 -> [w242 _ w249]
          frame 0, Default {
          }
          frame 1 {
            n172 = call "createSimpleArray.vi"("nbpoint1"=w244, "Bgstop"=w245, "Bgstart"=w246) -> ("Outarray"=w243:dbl[])
          }
          frame 2 {
            n173 = call "createSimpleArray.vi"("nbpoint1"=w250, "Bgstop"=w251, "Bgstart"=w252) -> ("Outarray"=w248:dbl[])
            n174 = Insert Into Array(array=w249, new element=w248) -> (w247:dbl[])  [unwired: 1 in]
          }
        }
        n175 = local write "Wavelength [nm]"(w235) -> ()
      }
      frame "mainLoop" {
        n176 = global write "stopButton.vi" "stopsignal"(FALSE) -> ()
        n177 = global write "GlobalVar.vi" "Set Persistent"("Set Persistent") -> ()
        n178 = local read "Total sweep sequence"() -> (w288:dbl[][])
        n179 = Index Array(array=w288, index (row)=0) -> (element=w271:dbl[])  [unwired: 1 in]
        "Num elements in col" <- w271
        n180 = local read "Device Cluster"() -> (w278:T4)
        n181 = local read "Loop Cluster"() -> (w287:T6)
        n182 = local read "Conversion Factor Sweep\n1 V = ??"() -> (w280:dbl)
        n183 = Array Size(array=w271) -> (size(s)=w273:i32)
        n184 = Array Size(array=w271) -> (size(s)=w293:i32)
        n185 = local read "Conversion Factor Fix\n1 V = ??"() -> (w279:dbl)
        n186 = Array Subset(array=w271, index=1) -> (w291:dbl[])  [unwired: 1 in]
        n187 = local read "Sweep Rate [T/min]"() -> (w260:dbl)
        n188 = Unbundle By Name(w287) -> ("Sweep Instrument"=w281:string, "Fix Instrument"=w254:string, "Wavelength"=w256:bool)  [unwired: 6 out]
        n189 = local read "Priority type array"() -> (w284:string[])
        n190 = local read "Gain Cluster 2"() -> (w286:T1)
        n191 = global read "GlobalVar.vi" "LaserControl"() -> (w255:T7)
        n192 = Array Size(array=w291) -> (size(s)=w295:i32)
        n193 = Unbundle By Name(w278) -> ("K2400 1"=w277:refnum<visa-resource-name>, "K2400 2"=w276:refnum<visa-resource-name>, "Lockin1"=w275:refnum<visa-resource-name>, "ITC signal"=w274:T2)
        n194 = Decrement(x=w273) -> (x-1=w272:i32)
        n195 = Initialize Array(1, w293) -> (→"row state":i32[])
        n196 = global write "GlobalVar.vi" "Sweep rate [T/min]"(w260) -> ()
        n197 = Bundle By Name(cluster=w255, "Power Stabilization"="Power stabilization") -> (w257:T7)
        n198 = while {
          tunnel: w295 -> [_]
          shift-right: [w343] -> _
          shift-left: "start" -> [w344]
          tunnel: w288 -> [w342]
          tunnel: w286 -> [w341]
          tunnel: w278 -> [w340]
          tunnel: w284 -> [w339]
          tunnel: [w323] -> w283
          tunnel: "init" -> [w338]
          tunnel: [w338] -> w268
          tunnel: w254 -> [w337]
          tunnel: w281 -> [w336]
          tunnel: w260 -> [w335]
          tunnel: w260 -> [w334]
          tunnel: w260 -> [w333]
          tunnel: w280 -> [w332]
          tunnel: w279 -> [w331]
          tunnel: w277 -> [w330]
          tunnel: w276 -> [w329]
          tunnel: w275 -> [w328]
          tunnel: w274 -> [w327]
          tunnel: [w322] -> w263
          tunnel: [w321] -> w262
          tunnel: [w320] -> w261
          tunnel: w256 -> [w319]
          tunnel: w255 -> [w318]
          tunnel: "Sweep Field back to zero" -> [_]
          stop <- w323 stop-if-true
          n199 = case shown="\"sweep\"" w344 {
            selector: w344 -> [_ _ _ w531]
            tunnel: ["sweep" w431 w486 w531] -> w343
            tunnel: w342 -> [w361 w433 w482 _]
            tunnel: [_ _ _ TRUE] -> w325
            tunnel: w341 -> [_ w425 _ _]
            tunnel: w340 -> [_ w424 _ _]
            tunnel: w339 -> [w360 w419 w481 _]
            tunnel: w337 -> [w358 w416 w480 _]
            tunnel: w336 -> [w359 w415 w479 _]
            tunnel: w335 -> [_ _ w478 _]
            tunnel: w334 -> [w357 _ _ _]
            tunnel: w333 -> [_ w414 _ _]
            tunnel: w332 -> [w356 w413 w476 _]
            tunnel: w331 -> [w355 w412 w477 _]
            tunnel: w330 -> [w352 w411 w472 _]
            tunnel: w329 -> [w353 w410 w473 _]
            tunnel: w328 -> [w351 w409 w474 _]
            tunnel: w327 -> [w354 w408 w475 _]
            tunnel: FALSE ("stopsignal") -> [_ w407 _ _]
            tunnel: [_ w403 _ _] -> w324
            tunnel: [_ w395 _ _] -> w322
            tunnel: [_ w394 _ _] -> w321
            tunnel: [_ w393 _ _] -> w320
            tunnel: w319 -> [w349 _ _ _]
            tunnel: w318 -> [w345 _ _ _]
            frame "start", Default {
              n200 = local read "Power stabilization"() -> (w348:bool)
              n201 = And(x=w349, y=w348) -> (x .and. y?=w347:bool)
              n202 = case shown="True" w347 {
                tunnel: [_ w369] -> w346
                tunnel: w345 -> [_ w366]
                frame False {
                }
                frame True {
                  n203 = global read "perHandlemonochromator.vi" "peHandle"() -> (w373:u32)
                  n204 = call "PE Get Wavelength.vi"("peHandle"=w373) -> ("error out"=w370:errorcluster, "wavelength"=w372:dbl)  [unwired: 8 in, 1 out]
                  n205 = call "GetPower.vi"("error in (no error)"=w370, "Wavelength (nm)"=w372, "Input Device"=refnum<visa-resource-name> "USB0::0x1313::0x8072::P2007928::INSTR") -> ("error out"=w369:errorcluster, "Power (W)"=w368:dbl)  [unwired: 1 in, 2 out]
                  n206 = Bundle By Name(cluster=w366, "Laser Power [W]"=w368) -> (w367:T7)
                  n207 = local write "Laser Power [W]"(w368) -> ()
                  n208 = global write "GlobalVar.vi" "LaserControl"(w367) -> ()
                }
              }
              n209 = local read "row state"() -> (w364:i32[])
              n210 = Array Size(array=w364) -> (size(s)=w363:i32)
              n211 = for {
                N: w363 -> [w390]
                tunnel: 1 -> [w391]
                tunnel: w361 -> [w392]
                tunnel: w360 -> [w386]
                tunnel: w359 -> [w384]
                tunnel: w358 -> [w383]
                tunnel: w357 -> [_]
                tunnel: w356 -> [w382]
                tunnel: w355 -> [w381]
                tunnel: w354 -> [w380]
                tunnel: w353 -> [w379]
                tunnel: w352 -> [w378]
                tunnel: w351 -> [w377]
                tunnel: [w376] -> _
                tunnel: [0 ("Current col")] -> w350
                tunnel: w346 -> [_]
                i -> [w389]
                n212 = Increment(x=w389) -> (x+1=w388:i32)
                n213 = Subtract(x=w390, y=w388) -> (x-y=w385:i32)
                n214 = Index Array(array=w386, index=w385) -> (element=w374:string)
                n215 = Index Array(array=w392, index (row)=w391, index (col)=w385) -> (element=w387:dbl)
                n216 = call "ApplyInstrument_v2.vi"("Instrument"=w374, "ITC ref"=w380, "Conversion Factor Fix\n1 V = ??"=w381, "K2400 1"=w378, "Sweep Instrument"=w384, "Valin"=w387, "Fix Instrument"=w383, "K2400 2"=w379, "Conversion Factor Sweep\n1 V = ??"=w382, "Lockin1"=w377) -> ("error out"=w376:errorcluster)  [unwired: 5 in]
              }
              n217 = local write "Current col"(w350) -> ()
            }
            frame "sweep" {
              w437 = 0 ("index")
              n218 = global write "stopButton.vi" "stopsignal"(w407) -> ()
              n219 = Index Array(array=w433, index (row)=w437, index (col)=w437) -> (element=w436:dbl)
              n220 = local read "counter"() -> (w398:i32)
              n221 = local read "File Basename"() -> (w422:string)
              n222 = local read "Folder Name"() -> (w423:path)
              n223 = local read "Current col"() -> (w417:i32)
              n224 = local read "row state"() -> (w430:i32[])
              n225 = local read "Refresh Rate [ms]"() -> (w404:i32)
              n226 = local read "Sweep Toothsaw"() -> (w396:bool)
              n227 = Quotient & Remainder(x=w398, y=2.0) -> (x-y*floor(x/y)=w400:dbl)  [unwired: 1 out]
              n228 = Index Array(array=w430, index=w417) -> (element=w434:i32)
              n229 = Not Equal To 0?(x=w400) -> (x != 0?=w397:bool)
              n230 = Index Array(array=w419, index=w417) -> (element=w418:string)
              n231 = call "autoNameFile.vi"("num"=w398, "File Basename"=w422, "Folder Name"=w423) -> ("path"=w426:path)
              n232 = Increment(x=w398) -> (x+1=w402:i32)
              n233 = for {
                N: w436 -> [_]
                tunnel: [w463] -> w431
                tunnel: "changerow" -> [w463]
                tunnel: w417 -> [w451]
                tunnel: w433 -> [w452]
                tunnel: [w451] -> w428
                shift-right: [w462] -> _
                shift-left: w434 -> [w450]
                tunnel: [TRUE] -> w421
                tunnel: w418 -> [w445]
                tunnel: [w440] -> _
                tunnel: w416 -> [w442]
                tunnel: w415 -> [w459]
                tunnel: w414 -> [_]
                tunnel: w413 -> [w458]
                tunnel: w412 -> [w457]
                tunnel: w411 -> [w444]
                tunnel: w410 -> [w443]
                tunnel: w409 -> [w456]
                tunnel: w408 -> [w455]
                tunnel: [w454] -> w403
                tunnel: [w453] -> _
                tunnel: w402 -> [w453]
                tunnel: [w453] -> w401
                tunnel: w397 -> [w449]
                tunnel: w396 -> [w446]
                tunnel: [w444] -> w395
                tunnel: [w443] -> w394
                tunnel: [w442] -> w393
                stop <- w454 stop-if-true
                n234 = And(x=w449, y=w446) -> (x .and. y?=w448:bool)
                n235 = Increment(x=w450) -> (x+1=w462:i32)
                n236 = case shown="True" w448 {
                  tunnel: w450 -> [w464 w467]
                  tunnel: w452 -> [_ w471]
                  tunnel: w451 -> [_ w469]
                  tunnel: [w464 w466] -> w447
                  frame False {
                    # "forth"
                  }
                  frame True {
                    n237 = Index Array(array=w471, index (row)=0, index (col)=w469) -> (element=w468:dbl)
                    n238 = Decrement(x=w467) -> (x-1=w465:i32)
                    n239 = Subtract(x=w468, y=w465) -> (x-y=w466:dbl)
                  }
                }
                n240 = global read "Visa name1.vi" "VISA name"() -> (w438:refnum<visa-resource-name>)
                n241 = Index Array(array=w452, index (row)=w447, index (col)=w451) -> (element=w460:dbl)
                n242 = local read "Step Delay (ms)"() -> (w439:dbl)
                n243 = call "ApplyInstrument_v2.vi"("Instrument"=w445, "ITC ref"=w455, "Conversion Factor Fix\n1 V = ??"=w457, "K2400 1"=w444, "Sweep Instrument"=w459, "Valin"=w460, "Fix Instrument"=w442, "DAC COM port"=w438, "K2400 2"=w443, "Conversion Factor Sweep\n1 V = ??"=w458, "Lockin1"=w456) -> ("error out"=w441:errorcluster)  [unwired: 4 in]
                n244 = local read "Cancel run"() -> (w454:bool)
                n245 = call "wait.vi"("error in (no error)"=w441, "wait time (ms)"=w439) -> ("error in (no error) 2"=w440:errorcluster)
              }
              n246 = local write "counter"(w402) -> ()
              n247 = call "gums_measureLoopV2.vi"("File Name"=w426, "SaveDataQuery"=TRUE, "Gain Cluster 2"=w425, "Refresh Rate [ms]"=w404, "Device Cluster"=w424) -> ()  [unwired: 6 in]
              n248 = local read "TotalPnts"() -> (w406:dbl)
              n249 = global write "stopButton.vi" "stopsignal"(w421) -> ()
              n250 = Divide(x=w401, y=w406) -> (x/y=w405:dbl)
              n251 = Increment(x=w428) -> (x+1=w432:i32)
              n252 = Replace Array Subset(array=w430, new element=1 ("new element/subarray"), index=w428) -> (w429:i32[])
              n253 = local write "Current col"(w432) -> ()
              n254 = local write "row state"(w429) -> ()
              n255 = local write "Total Progress"(w405) -> ()
            }
            frame "changerow" {
              n256 = local read "Current col"() -> (w483:i32)
              n257 = local read "row state"() -> (w493:i32[])
              n258 = local read "Num elements in col"() -> (w491:i32[])
              n259 = Index Array(array=w493, index=w483) -> (element=w489:i32)
              n260 = Array Size(array=w491) -> (size(s)=w490:i32)
              n261 = Index Array(array=w491, index=w483) -> (element=w496:i32)
              n262 = Increment(x=w489) -> (x+1=w488:i32)
              n263 = Greater?(x=w488, y=w496) -> (0:w495:bool)
              n264 = case shown="False" w495 {
                tunnel: [w519 0] -> w484
                tunnel: w488 -> [w519 _]
                tunnel: [w517 w525] -> w494
                tunnel: [w514 w522] -> w487
                tunnel: w483 -> [w518 w526]
                tunnel: w490 -> [_ w524]
                frame False {
                  n265 = Decrement(x=w518) -> (x-1=w517:i32)
                  n266 = Equal?(x=0, y=w517) -> (x = y?=w515:bool)
                  n267 = case shown="False" w515 {
                    tunnel: ["changerow" "sweep"] -> w514
                    frame False {
                    }
                    frame True {
                    }
                  }
                }
                frame True {
                  n268 = Increment(x=w526) -> (x+1=w525:i32)
                  n269 = Greater?(x=w525, y=w524) -> (0:w523:bool)
                  n270 = case shown="False" w523 {
                    tunnel: ["changerow" "stop"] -> w522
                    frame False {
                    }
                    frame True {
                    }
                  }
                }
              }
              n271 = local write "Current col"(w494) -> ()
              n272 = Replace Array Subset(array=w493, new element=w484, index=w483) -> (w492:i32[])
              n273 = Not Equal To 0?(x=w484) -> (x != 0?=w485:bool)
              n274 = case shown="True" w485 {
                tunnel: w487 -> [w497 w513]
                tunnel: [w497 w513] -> w486
                tunnel: w482 -> [_ w512]
                tunnel: w483 -> [_ w507]
                tunnel: w484 -> [_ w511]
                tunnel: w481 -> [_ w508]
                tunnel: w480 -> [_ w506]
                tunnel: w479 -> [_ w505]
                tunnel: w478 -> [_ _]
                tunnel: w477 -> [_ w504]
                tunnel: w476 -> [_ w503]
                tunnel: w475 -> [_ w502]
                tunnel: w474 -> [_ w501]
                tunnel: w473 -> [_ w500]
                tunnel: w472 -> [_ w499]
                frame False {
                }
                frame True {
                  n275 = Index Array(array=w512, index (row)=w511, index (col)=w507) -> (element=w509:dbl)
                  n276 = Index Array(array=w508, index=w507) -> (element=w498:string)
                  n277 = Wait (ms)(milliseconds to wait=u32 400) -> ()  [unwired: 1 out]
                  n278 = call "ApplyInstrument_v2.vi"("Instrument"=w498, "ITC ref"=w502, "Conversion Factor Fix\n1 V = ??"=w504, "K2400 1"=w499, "Sweep Instrument"=w505, "Valin"=w509, "Fix Instrument"=w506, "K2400 2"=w500, "Conversion Factor Sweep\n1 V = ??"=w503, "Lockin1"=w501) -> ()  [unwired: 5 in, 1 out]
                }
              }
              n279 = local write "row state"(w492) -> ()
            }
            frame "stop" {
            }
          }
          n280 = Or(x=w325, y=w324) -> (x .or. y?=w323:bool)
        }
        n281 = global write "GlobalVar.vi" "LaserControl"(w257) -> ()
        n282 = for {
          N: w272 -> [_]
          tunnel: w271 -> [w315]
          shift-right: [w312] -> w269
          shift-left: 1 ("index") -> [w313]
          i -> [w317]
          n283 = Increment(x=w317) -> (x+1=w316:i32)
          n284 = Index Array(array=w315, index=w316) -> (element=w314:dbl)
          n285 = Multiply(x=w313, y=w314) -> (x*y=w312:dbl)
        }
        "TotalPnts" <- w269
        n286 = case shown="True" "Sweep Field back to zero" {
          tunnel: w268 -> [w306 w311]
          tunnel: [w306 w311] -> w265
          frame False {
          }
          frame True {
            n287 = node("Zero ramp Rate [T/min] 2") -> (w310:dbl[unit])
            n288 = node(0.0) -> (w309:dbl[unit])
            n289 = call "TeslSetField.vi"("Sweep rate"=w310, "Field required:"=w309) -> ()  [unwired: 2 in, 2 out]
          }
        }
        n290 = Not(x=w283) -> (.not. x?=w267:bool)
        n291 = local write "START"(w267) -> ()
        n292 = global write "stopButton.vi" "stopsignal"(w267) -> ()
        n293 = local read "Sweep back\nto zero?"() -> (w266:bool)
        n294 = case shown="True" w266 {
          tunnel: w265 -> [w299 w305]
          tunnel: [w299 w305] -> w264
          tunnel: w263 -> [_ w302]
          tunnel: w262 -> [_ w301]
          tunnel: w261 -> [_ _]
          tunnel: w254 -> [_ w300]
          frame False {
          }
          frame True {
            n295 = call "ApplyInstrument_v2.vi"("Instrument"="Fixarray", "K2400 1"=w302, "Valin"=0.0, "Fix Instrument"=w300, "K2400 2"=w301) -> ()  [unwired: 10 in, 1 out]
          }
        }
        "Current col" <- -1 ("Current col")
        "counter" <- 0 ("counter")
      }
      frame "loopIncrease" {
        w544 = 1 ("Nb Sweep Indicator")
        # "VERIFY IF THIS IS REALLY NECESSARY\n14.10.2020"
        n296 = local read "Nb Loop Indicator"() -> (w547:i32)
        n297 = local read "sweep stop 2 [V]"() -> (w540:dbl)
        n298 = local read "sweep stop [V]"() -> (w542:dbl)
        n299 = local read "Nb steps 2"() -> (w539:i32)
        n300 = local read "Nb steps"() -> (w538:i32)
        n301 = Add(x=w540, y="Gate Increase 2 (V)") -> (x+y=w532:dbl)
        n302 = Add(x="Gate Increase (V)", y=w542) -> (x+y=w533:dbl)
        n303 = Add(x="Nb steps Increase", y=w538) -> (x+y=w534:dbl)
        n304 = Add(x="Nb steps Increase 2", y=w539) -> (x+y=w535:dbl)
        n305 = Increment(x=w547) -> (x+1=w546:i32)
        n306 = local write "sweep stop 2 [V]"(w532) -> ()
        n307 = local write "sweep stop [V]"(w533) -> ()
        n308 = local write "Nb steps"(w534) -> ()
        n309 = local write "Nb Loop Indicator"(w546) -> ()
        n310 = local write "Nb steps 2"(w535) -> ()
        n311 = local write "Priority B"(w544) -> ()
        n312 = local write "Nb Sweep Indicator"(w544) -> ()
      }
      frame "endRun" {
        n313 = local read "Device Cluster"() -> (w549:T4)
        n314 = case shown="True" "Sweep back to zero" {
          frame False {
          }
          frame True {
            n315 = call "K2400_ApplyVOLTsafe_GUMS.vi"("Voltage target [V]"=0.0) -> ()  [unwired: 2 in]
          }
        }
        n316 = Unbundle By Name(w549) -> ("DAC present"=w548:bool)
        n317 = case shown="True" w548 {
          frame False {
          }
          frame True {
            n318 = local read "DAC"() -> (w553:refnum<visa-resource-name>)
            n319 = call "closeRS232.vi"("VISA resource name"=w553) -> ()  [unwired: 2 in]
          }
        }
      }
      frame "EmptyArrays" {
        w556 = 0.0
        n320 = Initialize Array(w556, w556) -> (w555:dbl[])
        n321 = local write "B [T]"(w555) -> ()
        n322 = local write "T [K]"(w555) -> ()
        n323 = local write "Sweep Bias"(w555) -> ()
        n324 = local write "Fix Bias"(w555) -> ()
      }
      frame "DACioload" {
        n325 = local read "DACindic"() -> (w560:bool)
        n326 = local read "DAC"() -> (w561:refnum<visa-resource-name>)
        n327 = case shown="True" w560 {
          tunnel: w561 -> [w563 w565]
          tunnel: "init" -> [w562 w564]
          tunnel: [w562 w564] -> w558
          frame False {
            n328 = call "closeRS232.vi"("VISA resource name"=w563) -> ()  [unwired: 2 in]
          }
          frame True {
            n329 = call "openRS232.vi"("com"=w565) -> ("VISA resource name"=w566:refnum<visa-resource-name>)  [unwired: 1 out]
            n330 = global write "Visa name1.vi" "VISA name"(w566) -> ()
          }
        }
      }
      frame "FCprocedure" {
        n331 = while {
          tunnel: "init" -> [w574]
          tunnel: [w574] -> w567
          shift-right: [w572] -> _
          shift-left: "setfield" -> [w575]
          tunnel: [FALSE] -> w568
          stop <- w573 stop-if-true
          n332 = case shown="\"gumsIT\"" w575 {
            tunnel: [TRUE _ _ _ _ _] -> w573
            tunnel: ["" w587 "wait" "RampField2Zero" w612 w629] -> w572
            frame "out", Default {
              n333 = global write "stopButton.vi" "stopsignal"(FALSE) -> ()
              n334 = local write "I am"("finished") -> ()
            }
            frame "setfield" {
              n335 = local read "counter 2"() -> (w581:i32)
              n336 = local read "Bipolar"() -> (w582:bool)
              n337 = Greater Than 0?(x=w581) -> (x > 0?=w580:bool)
              n338 = local read "Cooling field (T)"() -> (w585:dbl)
              n339 = local write "I am"("Ramping the field up") -> ()
              n340 = And(x=w582, y=w580) -> (x .and. y?=w583:bool)
              n341 = case shown="True" w583 {
                tunnel: [w593 w594] -> w584
                tunnel: w585 -> [w593 w596]
                frame False {
                }
                frame True {
                  n342 = Multiply(x=w596, y=-1.0) -> (x*y=w594:dbl)
                }
              }
              n343 = local read "sweep rate B (T/min)"() -> (w590:dbl)
              n344 = node(w590) -> (w589:dbl[unit])
              n345 = node(w584) -> (w591:dbl[unit])
              n346 = call "TeslSetField.vi"("Set Persistent"=TRUE, "Sweep rate"=w589, "Field required:"=w591) -> ("OK?"=w588:bool)  [unwired: 1 in, 1 out]
              n347 = case shown="False" w588 {
                selector: w588 -> [w598 w599]
                tunnel: ["out" "cooldown"] -> w587
                frame False {
                  n348 = local write "Field ok !"(w598) -> ()
                }
                frame True {
                  "Field ok !" <- w599
                }
              }
            }
            frame "cooldown" {
              n349 = local read "Base T (K)"() -> (w601:dbl)
              n350 = local read "ITC ref"() -> (w603:T2)
              n351 = call "Tloop.vi"("ITCSignal"=w603, "T target [K]"=w601, "Regulate ?"=TRUE) -> ()  [unwired: 2 in, 2 out]
              n352 = local write "I am"("Cooling down to base T") -> ()
            }
            frame "wait" {
              n353 = local read "Waiting time (min)"() -> (w608:dbl)
              n354 = local write "I am"("Waiting") -> ()
              n355 = Multiply(x=w608, y=60000.0) -> (x*y=w610:dbl)
              n356 = Wait (ms)(milliseconds to wait=w610) -> ()  [unwired: 1 out]
            }
            frame "RampField2Zero" {
              n357 = local read "sweep rate B (T/min)"() -> (w616:dbl)
              n358 = node(w616) -> (w617:dbl[unit])
              n359 = local write "I am"("Ramping the field back to zero") -> ()
              n360 = call "TeslSetField.vi"("Set Persistent"=TRUE, "Sweep rate"=w617, "Field required:"=dbl[unit] 0.0) -> ()  [unwired: 1 in, 2 out]
              n361 = case shown="False" FALSE {
                tunnel: ["gumsIT" "degauss"] -> w612
                frame False {
                }
                frame True {
                  # "To be done"
                }
              }
            }
            frame "gumsIT" {
              n362 = global write "stopButton.vi" "stopsignal"(FALSE) -> ()
              n363 = local read "Temperature Up rate (K/min)"() -> (w626:dbl)
              n364 = local read "High T (K)"() -> (w627:dbl)
              n365 = local read "Base T (K)"() -> (w628:dbl)
              n366 = local read "ITC ref"() -> (w625:T2)
              n367 = local read "File Basename"() -> (w637:string)
              n368 = local read "Folder Name"() -> (w636:path)
              n369 = local read "counter 2"() -> (w624:i32)
              n370 = local read "Bipolar"() -> (w630:bool)
              n371 = call "Tloop.vi"("ITCSignal"=w625, "T target [K]"=w628, "Precision"=w627, "Time limit"=w626) -> ("ITCSignal 2"=w623:T2, "Finish"=w622:bool)  [unwired: 1 in]
              n372 = local read "Refresh Rate [ms]"() -> (w631:i32)
              n373 = local read "Device Cluster"() -> (w632:T4)
              n374 = local read "Gain Cluster 2"() -> (w633:T1)
              n375 = local write "I am"("Heating up and acquiring hopefully amazing data") -> ()
              n376 = case shown="True" w630 {
                tunnel: w624 -> [_ w643]
                tunnel: ["out" w639] -> w629
                tunnel: w623 -> [_ _]
                frame False {
                }
                frame True {
                  n377 = Increment(x=w643) -> (x+1=w640:i32)
                  n378 = local write "counter 2"(w640) -> ()
                  n379 = Greater?(x=w640, y=1) -> (0:w642:bool)
                  n380 = case shown="True" w642 {
                    tunnel: w640 -> [w645 w647]
                    tunnel: [w645 w647] -> _
                    tunnel: ["setfield" "out"] -> w639
                    frame False {
                    }
                    frame True {
                    }
                  }
                }
              }
              n381 = global write "stopButton.vi" "stopsignal"(w622) -> ()
              n382 = call "autoNameFile.vi"("num"=w624, "File Basename"=w637, "Folder Name"=w636) -> ("path"=w635:path)
              n383 = call "gums_measureLoopV2.vi"("File Name"=w635, "SaveDataQuery"=TRUE, "Gain Cluster 2"=w633, "Refresh Rate [ms]"=w631, "Device Cluster"=w632) -> ()  [unwired: 6 in]
            }
          }
        }
        n384 = local write "START FC"(w568) -> ()
      }
    }
    "x .or. y?" <- w27
  }
  n385 = Unbundle By Name("Gain Cluster 2") -> ("conversion factor BG"=→"conversion factor sweep":dbl, "Vin / Vout 1"=→"Bias factor":dbl)  [unwired: 10 out]
  n386 = Unbundle By Name("Device Cluster") -> ("K2400 1"=→"K2400 1":refnum<visa-resource-name>, "Lockin1"=→"Lockin1":refnum<visa-resource-name>, "K2400 2"=→"K2400 2":refnum<visa-resource-name>, "DAC"=w3:refnum<visa-resource-name>, "ITC signal"=→"ITC ref":T2, "DAC present"=w4:bool, "DMMX"=→"DMMX":string[][])  [unwired: 3 out]
  "DAC" <- w3
  n387 = case shown="True" w4 {
    tunnel: w3 -> [_ w648]
    frame False {
    }
    frame True {
      n388 = call "openRS232.vi"("com"=w648) -> ("VISA resource name"=w649:refnum<visa-resource-name>)  [unwired: 1 out]
      n389 = global write "Visa name1.vi" "VISA name"(w649) -> ()
    }
  }
  "Nb Sweep Indicator" <- 1 ("Nb Sweep Indicator")
  "Nb Loop Indicator" <- 0.0 ("Nb Sweep Indicator")
